vi "subdev spec make.vi"(8 "error in (no error)":errorcluster, 10 "markup":string, 11 "h":u64) -> (0 "error out":errorcluster, 2 "function return":u32(ring), 3 "h out":u64)   [LabVIEW 2023, in "uhd.lvlib"]
doc: "UHD_API uhd_error uhd_subdev_spec_make(uhd_subdev_spec_handle* h, const char* markup);"
uses:
  <userlib>/uhd/uhd.lvlib
  <userlib>/uhd/uhd.dll
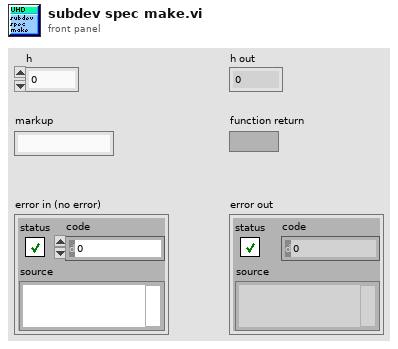
[diagram p1: front panel]
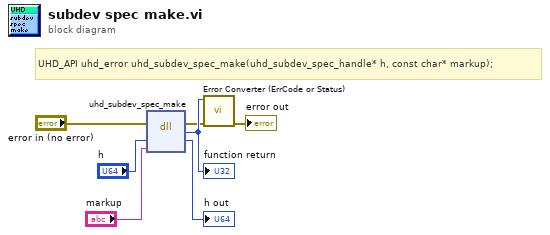
[diagram p0: block diagram]
diagram:
  # "UHD_API uhd_error uhd_subdev_spec_make(uhd_subdev_spec_handle* h, const char* markup);"
  n1 = dll-call lib="C:/Program Files/National Instruments/LabVIEW 2023/user.lib/uhd/uhd.*" fn="uhd_subdev_spec_make"(error in="error in (no error)", "h"="h", "markup"="markup") -> (error out=w2:errorcluster, w7:u32, "h"=→"h out":u64)  [unwired: 3 in, 1 out]
  "function return" <- w7
  n2 = call <userlib>:"Error Converter (ErrCode or Status).vi"("error in (no error)"=w2, "error code"=w7) -> ("error out"=→"error out":errorcluster)  [unwired: 9 in]
